vi "CreateMemoryNode.vi"(7 "DOM Document":refnum<k20>, 8 "Error In":errorcluster, 11 "Memory":string[](array[string])) -> (0 "Error Out":errorcluster, 3 "Memory Node":refnum<k20>)   [LabVIEW 2012]
uses:
  libs/LV-Utilities/LV-Utilities.lvlib
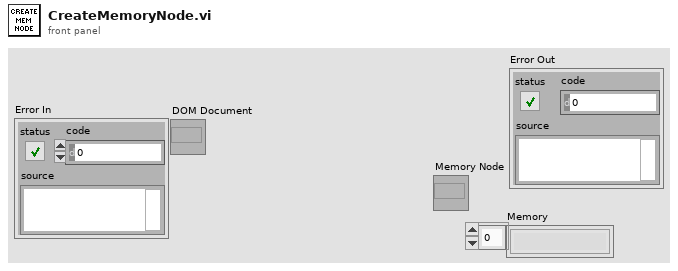
[diagram p1: front panel]
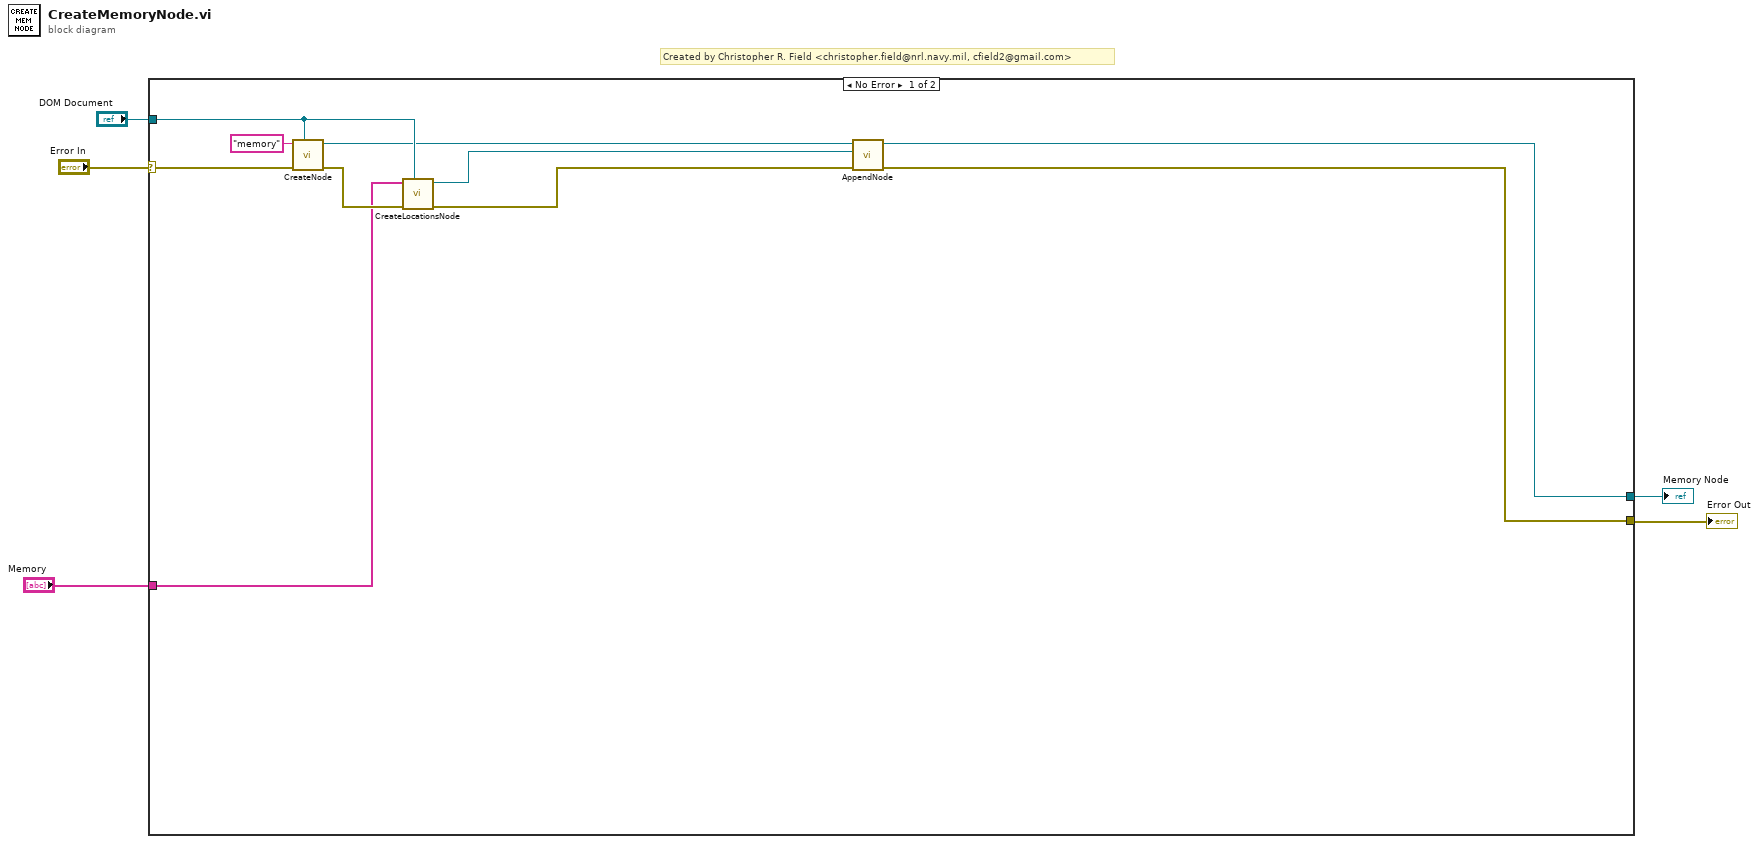
[diagram p0: block diagram]
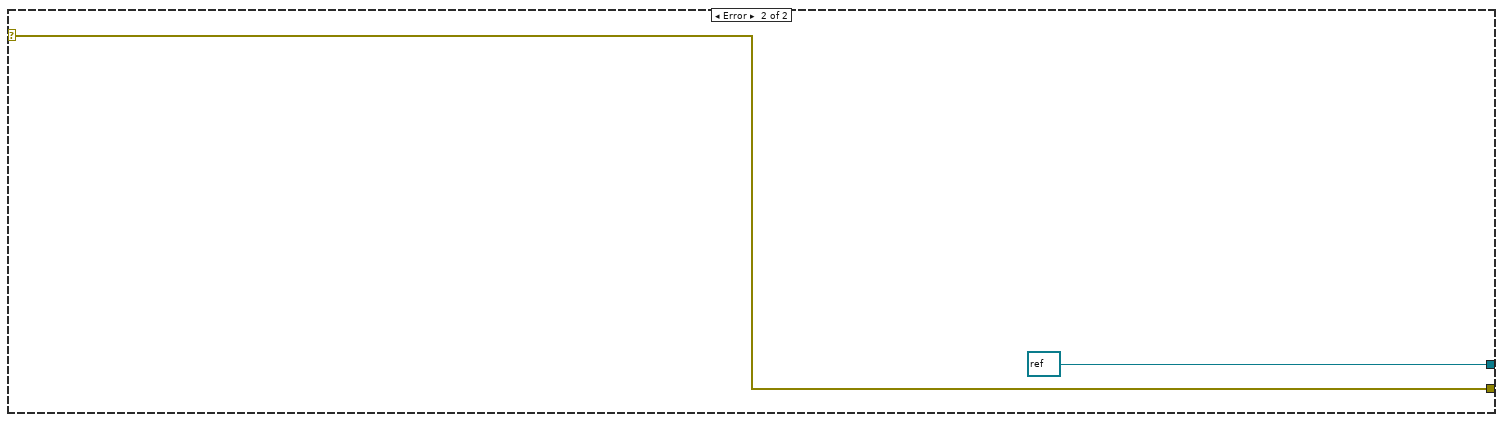
[diagram p2: hidden frame]
diagram:
  # "Created by Christopher R. Field <christopher.field@nrl.navy.mil, cfield2@gmail.com>"
  n1 = case shown="No Error" "Error In" {
    selector: "Error In" -> [w15 w17]
    tunnel: "DOM Document" -> [w11 _]
    tunnel: [w12 w17] -> w3
    tunnel: [w13 refnum<k20> refnum ("Wirings Node 2")] -> w2
    tunnel: "Memory" -> [w9 _]
    frame No Error {
      n2 = call "CreateNode.vi"("DOM Document"=w11, "Error In"=w15, "Tag Name"="memory") -> ("Error out"=w10:errorcluster, "Node"=w6:refnum<k20>)  [unwired: 7 in]
      n3 = call "CreateLocationsNode.vi"("DOM Document"=w11, "Error In"=w10, "Memory"=w9) -> ("Error Out"=w8:errorcluster, "Locations Node"=w7:refnum<k20>)  [unwired: 7 in]
      n4 = call "AppendNode.vi"("Error In"=w8, "Child Node"=w7, "Parent Node In"=w6) -> ("Error Out"=w12:errorcluster, "Parent Node Out"=w13:refnum<k20>)  [unwired: 7 in]
    }
    frame Error {
    }
  }
  "Memory Node" <- w2
  "Error Out" <- w3
